vi "Send Menu Selection (User).vi"(7 "Message Priority (Normal)":T1=enum."Normal", 8 "error in (no error)":errorcluster, 9 "ItemPath":string, 10 "ItemTag":string, 11 "Message Enqueuer":refnum<class "Message Enqueuer.lvclass">) -> (0 "error out":errorcluster, 3 "Message Enqueuer out":refnum<class "Message Enqueuer.lvclass">)   [LabVIEW 2021, in "Shortcut Menu.lvlib" / "Menu Selection (User) Msg.lvclass"]
doc: "This VI sends the message to an actor."
uses:
  <userlib>/John_Lib/Interfaces/Shortcut Menu Messages/Menu Selection (User) Msg/Menu Selection (User) Msg.lvclass
  <vilib>/ActorFramework/Message Enqueuer/Message Enqueuer.lvclass
  <vilib>/ActorFramework/Message Enqueuer/Message Priority.ctl
  C:/Program Files (x86)/National Instruments/LabVIEW 2021/vi.lib/ActorFramework/Message/Message.lvclass
  <userlib>/John_Lib/Interfaces/Shortcut Menu Messages/Menu Selection (User) Msg/Menu Selection (User) Msg.lvclass/Menu Selection (User) Msg.ctl
  <vilib>/ActorFramework/Message Enqueuer/Message Enqueuer.lvclass/Message Enqueuer.ctl
  <vilib>/ActorFramework/Message Priority Queue/Priority Enqueue.vi
  C:/Program Files (x86)/National Instruments/LabVIEW 2021/user.lib/John_Lib/Interfaces/Shortcut Menu Messages/Menu Selection (User) Msg/Menu Selection (User) Msg.lvclass
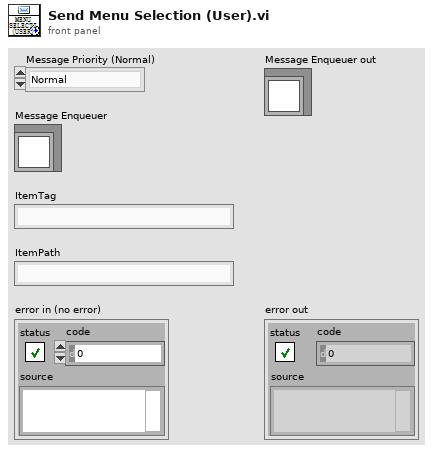
[diagram p1: front panel]
types:
  T1 = typedef "Actor Framework.lvlib/Message Enqueuer.lvclass/Message Priority.ctl" = enum16{"Low", "Normal", "High"}
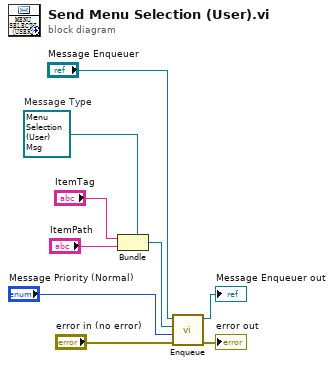
[diagram p0: block diagram]
diagram:
  w6 = refnum<class "Menu Selection (User) Msg.lvclass"> refnum  # Message Type
  n1 = Bundle(cluster=w6, "ItemTag", "ItemPath") -> (w5:refnum<class "Menu Selection (User) Msg.lvclass">)
  n2 = call <vilib>:"Enqueue.vi"("error in (no error)"="error in (no error)", "Message Priority (Normal)"="Message Priority (Normal)", "Message"=w5, "Message Enqueuer in"="Message Enqueuer") -> ("error out"=→"error out":errorcluster, "Message Enqueuer in"=→"Message Enqueuer out":refnum<class "Message Enqueuer.lvclass">)  [unwired: 6 in]
